vi "SQLHistorylab.vi"() -> ()   [LabVIEW 2013]
uses:
  <vilib>/Platform/TimedLoop/XDataNode/timing_clust.ctl
  <vilib>/Platform/TimedLoop/XDataNode/nitl_modes.ctl
  <vilib>/Platform/TimedLoop/XDataNode/wakeup.ctl
  <vilib>/platform/TimedLoop/XDataNode/XDataNode.xnode
  <vilib>/Platform/TimedLoop/XDataNode/XDNodeRunTimeDep.lvlib
panel:
  out "SSE PV":string
  out "BL13-2SPECPV":string
  out "HIROHITO1PC":T1(plugin-control)
  out "BL13-2DVMPV":string
  out "decimal integer string":string
  out "time string":string
  out "date string":string
  out "CAM2":T1(plugin-control)
  out "CAM1":T1(plugin-control)
  out "CAM3":T1(plugin-control)
  in  "13-2SPEC PV":bool
  out "PV2ELOG":string
  in  "Author":string
  in  "Subject":string
  out "concatenated string":string
  out "standard error":string
  out "standard output":string
  in  "Path":path
  in  "Logbook":u16(ring) items=["BL13-2", "BL13-2 APPES", "BL13-2 SSE"]
  in  "Attachment":bool
  in  "Cam5":bool
  in  "Cam4":bool
  in  "Cam3":bool
  in  "Cam2":bool
  in  "Cam1":bool
  in  "R3000/XES PV":bool
  in  "SES-100PV":bool
  in  "SSE PV":bool
  in  "APPES  PV":bool
  in  "13-2DVM PV":bool
  in  "Submit":bool
  in  "stop":bool
  in  "ELOG":string
  # "BL13-2 ELOG"
  # "[PV name] [PV value] [Time]"
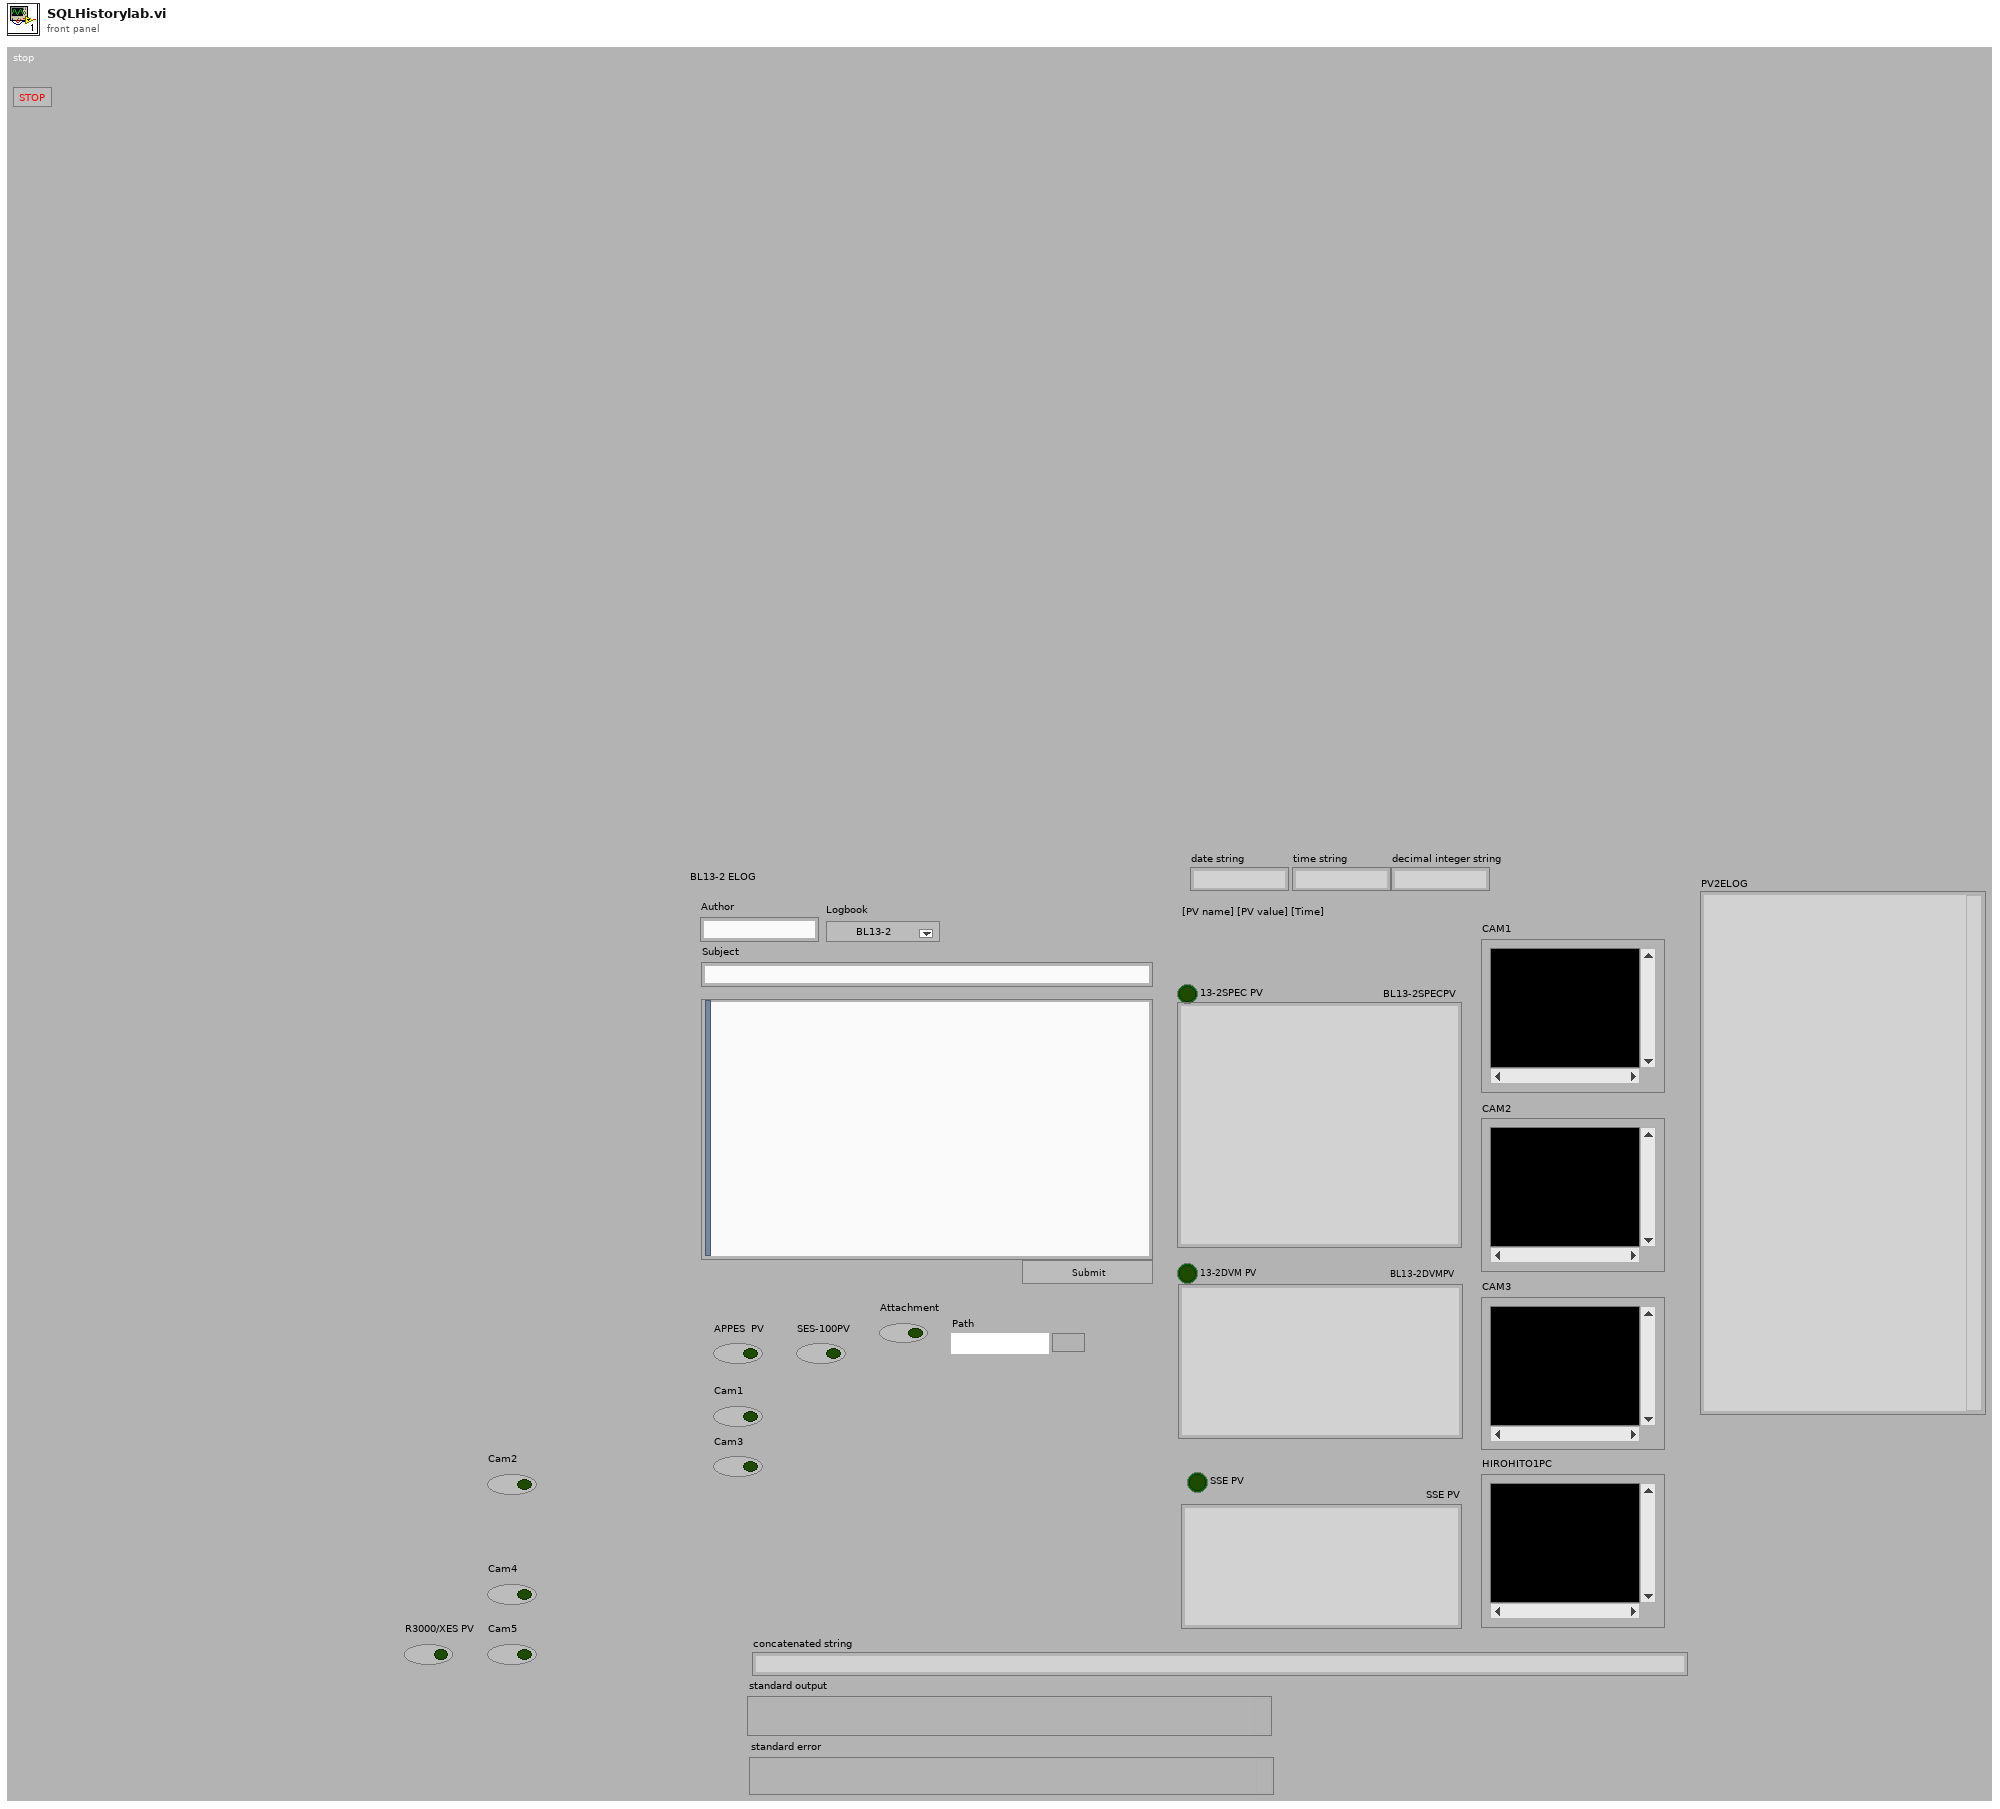
[diagram p1: front panel]
types:
  T1 = typedef "IMAQ Image.ctl" = refnum<image>
  T2 = typedef "XDNodeRunTimeDep.lvlib/timing_clust.ctl" = cluster{"Expected End [f-1]":u64, "Actual End [f-1]":u64, "Finished Late? [f-1]":bool, "Expected End [i-1]":u64, "Actual End [i-1]":u64, "Finished Late? [i-1]":bool, "Expected Start [i]":u64, "Actual Start [i]":u64, "Expected Start [f]":u64, "Actual Start [f]":u64, "Source Name":string, "Structure Name":string, "Period":i64, "Deadline":i64, "Offset":i64, "Start":i64, "Priority":i32, "Timeout":i32, "Mode":T3, "Wakeup Reason":T4, "Error":errorcluster, "Source Type":string, "Secondary Source Type":string, "Global End Time":u64, "Global Start Time":u64, "Frame Duration":u64, "Iteration Duration":u64, "Assigned CPU":i32, "I/O Scan Engine Mode":u32}
  T3 = typedef "XDNodeRunTimeDep.lvlib/nitl_modes.ctl" = enum32{"No Change", "Process missed periods, maintain original phase", "Discard missed periods, maintain original phase", "Process missed periods, ignore original phase", "Discard missed periods, ignore original phase"}
  T4 = typedef "XDNodeRunTimeDep.lvlib/wakeup.ctl" = enum32{"Normal", "Aborted", "Asynchronous wakeup", "Timing source error", "Timed loop error", "Timeout"}
  T5 = enum16{"open", "replace", "create", "open or create", "replace or create", "replace or create with confirmation"}
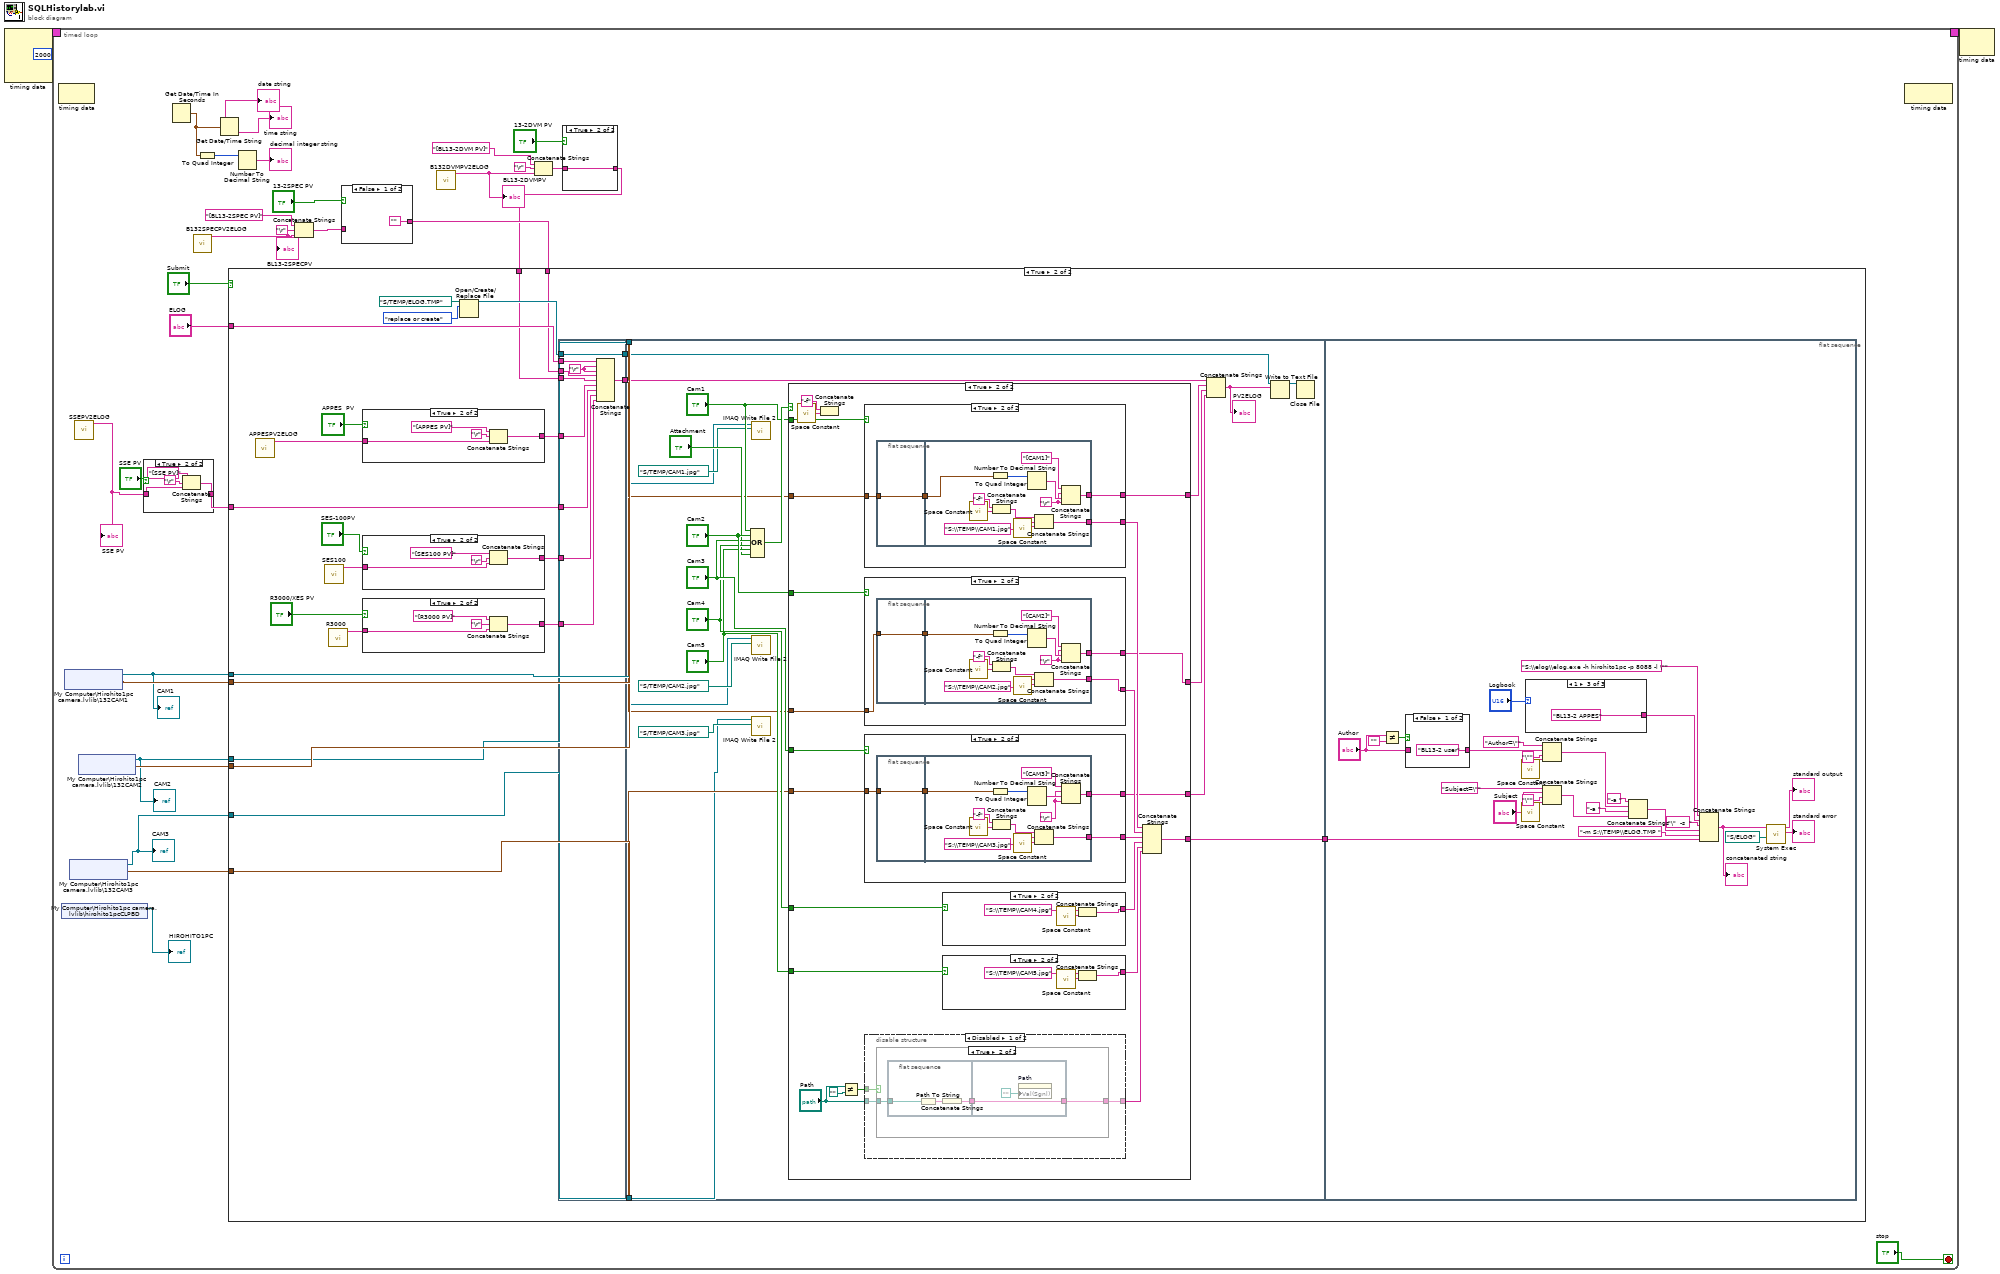
[diagram p0: block diagram]
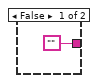
[diagram p2: hidden frame]
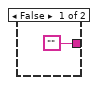
[diagram p3: hidden frame]
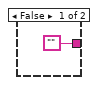
[diagram p6: hidden frame]
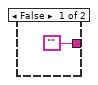
[diagram p7: hidden frame]
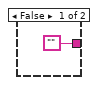
[diagram p8: hidden frame]
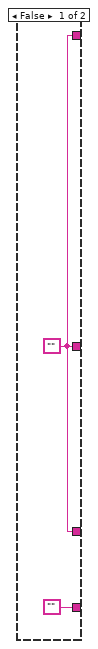
[diagram p9: hidden frame]
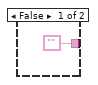
[diagram p10: hidden frame]
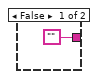
[diagram p12: hidden frame]
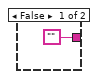
[diagram p13: hidden frame]
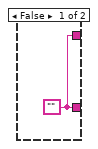
[diagram p14: hidden frame]
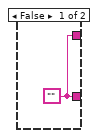
[diagram p15: hidden frame]
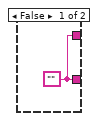
[diagram p16: hidden frame]
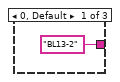
[diagram p18: hidden frame]
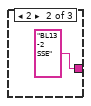
[diagram p19: hidden frame]
diagram:
  n1 = node-c288(i64 2000 ("Period")) -> (w3:T2)  [unwired: 3 in]
  n2 = timed-loop {
    timing: w3 -> [_]
    timing-out: [_] -> w2
    stop <- "stop" stop-if-true
    n3 = node-c288() -> ()  [unwired: 1 in, 1 out]
    n4 = shared-variable "My Computer\\Hirohito1pc camera.lvlib\\hirohito1pcCLPBD"() -> (→"HIROHITO1PC":refnum<image>)  [unwired: 1 in, 1 out]
    n5 = shared-variable "My Computer\\Hirohito1pc camera.lvlib\\132CAM1"() -> (w13:refnum<image>, w14:timestamp)  [unwired: 1 in, 1 out]
    "CAM1" <- w13
    n6 = shared-variable "My Computer\\Hirohito1pc camera.lvlib\\132CAM3"() -> (w9:refnum<image>, w10:timestamp)  [unwired: 1 in, 1 out]
    "CAM3" <- w9
    n7 = call "SSEPV2ELOG.vi"() -> ("concatenated string"=w4:string)  [unwired: 11 in]
    "SSE PV" <- w4
    n8 = shared-variable "My Computer\\Hirohito1pc camera.lvlib\\132CAM2"() -> (w11:refnum<image>, w12:timestamp)  [unwired: 1 in, 1 out]
    "CAM2" <- w11
    n9 = case shown="True" "SSE PV" {
      tunnel: ["" w36] -> w5
      tunnel: w4 -> [_ w37]
      frame False {
      }
      frame True {
        n10 = Concatenate Strings("[SSE PV]" ("string"), "\r", w37) -> (w36:string)
      }
    }
    n11 = Get Date/Time In Seconds() -> (seconds since 1Jan1904=w26:timestamp)
    n12 = call "B132SPECPV2ELOG.vi"() -> ("concatenated string"=w25:string)  [unwired: 11 in]
    "BL13-2SPECPV" <- w25
    n13 = To Quad Integer(1:w26) -> (0:w28:i64)
    n14 = Get Date/Time String(seconds (now)=w26) -> (date string=→"date string":string, time string=→"time string":string)  [unwired: 2 in]
    n15 = Number To Decimal String(number=w28) -> (decimal integer string=→"decimal integer string":string)  [unwired: 1 in]
    n16 = Concatenate Strings("[BL13-2SPEC PV]" ("string"), "\r", w25) -> (w24:string)
    n17 = case shown="False" "13-2SPEC PV" {
      tunnel: ["" w42] -> w20
      tunnel: w24 -> [_ w42]
      frame False {
      }
      frame True {
      }
    }
    n18 = call "B132DVMPV2ELOG.vi"() -> ("concatenated string 2"=w7:string)  [unwired: 11 in]
    "BL13-2DVMPV" <- w7
    n19 = Concatenate Strings("[BL13-2DVM PV]" ("string"), "\r", w7) -> (w19:string)
    n20 = case shown="True" "13-2DVM PV" {
      tunnel: ["" w40] -> w15
      tunnel: w19 -> [_ w40]
      frame False {
      }
      frame True {
      }
    }
    n21 = case shown="True" "Submit" {
      tunnel: "ELOG" -> [_ w69]
      tunnel: w20 -> [_ w53]
      tunnel: w15 -> [_ w52]
      tunnel: w14 -> [_ w51]
      tunnel: w13 -> [_ w50]
      tunnel: w12 -> [_ w49]
      tunnel: w11 -> [_ w48]
      tunnel: w10 -> [_ w47]
      tunnel: w9 -> [_ w46]
      tunnel: w5 -> [_ w45]
      frame False {
      }
      frame True {
        n22 = call "APPESPV2ELOG.vi"() -> ("concatenated string"=w56:string)  [unwired: 11 in]
        n23 = call "SES100.vi"() -> ("text"=w55:string)  [unwired: 11 in]
        n24 = call "R3000.vi"() -> ("text"=w54:string)  [unwired: 11 in]
        n25 = case shown="True" "APPES  PV" {
          tunnel: ["" w82] -> w65
          tunnel: w56 -> [_ w81]
          frame False {
          }
          frame True {
            n26 = Concatenate Strings("[APPES PV]" ("string"), "\r", w81) -> (w82:string)
          }
        }
        n27 = case shown="True" "SES-100PV" {
          tunnel: ["" w79] -> w61
          tunnel: w55 -> [_ w76]
          frame False {
          }
          frame True {
            n28 = Concatenate Strings("[SES100 PV]" ("string"), "\r", w76) -> (w79:string)
          }
        }
        n29 = case shown="True" "R3000/XES PV" {
          tunnel: ["" w74] -> w60
          tunnel: w54 -> [_ w71]
          frame False {
          }
          frame True {
            n30 = Concatenate Strings("[R3000 PV]" ("string"), "\r", w71) -> (w74:string)
          }
        }
        n31 = Open/Create/Replace File(file path (use dialog)=path "S:/TEMP/ELOG.TMP", operation (0:open)=T5."replace or create") -> (refnum out=w66:refnum<file>)  [unwired: 4 in, 2 out]
        n32 = flat-sequence {
          tunnel: w66 -> [w92]
          tunnel: w69 -> [w94]
          tunnel: w52 -> [w89]
          tunnel: w65 -> [w85]
          tunnel: w45 -> [w88]
          tunnel: w61 -> [w87]
          tunnel: w60 -> [w86]
          tunnel: w53 -> [w90]
          tunnel: [w92] -> w59
          tunnel: [w91] -> w58
          tunnel: w59 -> [w95]
          tunnel: w58 -> [w108]
          tunnel: [w105] -> w57
          tunnel: w51 -> [w101]
          tunnel: w50 -> [w100]
          tunnel: w49 -> [w99]
          tunnel: w48 -> [w98]
          tunnel: w47 -> [w97]
          tunnel: w46 -> [w96]
          tunnel: w57 -> [w220]
          frame #0 {
            w93 = "\r"
            n33 = Concatenate Strings(w94, w93, w93, w90, w89, w85, w88, w87, w86) -> (w91:string)
          }
          frame #1 {
            n34 = Compound Arithmetic op=OR("Cam1", "Cam2", "Cam3", "Cam4", "Cam5", "Attachment") -> (w118:bool)
            n35 = call-poly "IMAQ Write File 2"("File Path"=path "S:/TEMP/CAM1.jpg", "Image"=w100) -> ()  [unwired: 8 in, 2 out]
            n36 = call-poly "IMAQ Write File 2"("File Path"=path "S:/TEMP/CAM2.jpg", "Image"=w98) -> ()  [unwired: 8 in, 2 out]
            n37 = call-poly "IMAQ Write File 2"("File Path"=path "S:/TEMP/CAM3.jpg", "Image"=w96) -> ()  [unwired: 8 in, 2 out]
            n38 = case shown="True" w118 {
              tunnel: ["" w131] -> w105
              tunnel: "Cam1" -> [_ w136]
              tunnel: "Cam2" -> [_ w135]
              tunnel: "Cam3" -> [_ w134]
              tunnel: "Cam4" -> [_ w133]
              tunnel: "Cam5" -> [_ w132]
              tunnel: [w119 w129] -> w109
              tunnel: [w119 w128] -> w107
              tunnel: [w119 w127] -> w106
              tunnel: w101 -> [_ w123]
              tunnel: w99 -> [_ w122]
              tunnel: w97 -> [_ w121]
              frame False {
                w119 = ""
              }
              frame True {
                n39 = call <vilib>:"Space Constant.vi"() -> ("String"=w142:string)
                n40 = Concatenate Strings("-f", w142) -> ()  [unwired: 1 out]
                n41 = Not Equal?(x="Path", y=path "") -> (x != y?=w125:bool)
                n42 = case shown="True" w136 {
                  tunnel: [w200 w204] -> w141
                  tunnel: [w200 w203] -> w128
                  tunnel: w123 -> [_ w202]
                  frame False {
                    w200 = ""
                  }
                  frame True {
                    n43 = flat-sequence {
                      tunnel: w202 -> [w205]
                      tunnel: [w205] -> w201
                      tunnel: [w215] -> w204
                      tunnel: [w209] -> w203
                      tunnel: w201 -> [w210]
                      frame #0 {
                      }
                      frame #1 {
                        w211 = "\r"
                        n44 = call <vilib>:"Space Constant.vi"() -> ("String"=w207:string)
                        n45 = To Quad Integer(1:w210) -> (0:w214:i64)
                        n46 = Concatenate Strings("-f", w207) -> (w206:string)
                        n47 = call <vilib>:"Space Constant.vi"() -> ("String"=w216:string)
                        n48 = Number To Decimal String(number=w214) -> (decimal integer string=w212:string)  [unwired: 1 in]
                        n49 = Concatenate Strings(w206, "S:\\TEMP\\CAM1.jpg", w216) -> (w215:string)
                        n50 = Concatenate Strings("[CAM1]" ("string"), w211, w212, w211) -> (w209:string)
                      }
                    }
                  }
                }
                n51 = case shown="True" w135 {
                  tunnel: [w182 w186] -> w140
                  tunnel: [w182 w185] -> w127
                  tunnel: w122 -> [_ w184]
                  frame False {
                    w182 = ""
                  }
                  frame True {
                    n52 = flat-sequence {
                      tunnel: w184 -> [w187]
                      tunnel: [w187] -> w183
                      tunnel: [w197] -> w186
                      tunnel: [w191] -> w185
                      tunnel: w183 -> [w194]
                      frame #0 {
                      }
                      frame #1 {
                        w192 = "\r"
                        n53 = call <vilib>:"Space Constant.vi"() -> ("String"=w189:string)
                        n54 = To Quad Integer(1:w194) -> (0:w195:i64)
                        n55 = Concatenate Strings("-f", w189) -> (w188:string)
                        n56 = call <vilib>:"Space Constant.vi"() -> ("String"=w198:string)
                        n57 = Number To Decimal String(number=w195) -> (decimal integer string=w193:string)  [unwired: 1 in]
                        n58 = Concatenate Strings(w188, "S:\\TEMP\\CAM2.jpg", w198) -> (w197:string)
                        n59 = Concatenate Strings("[CAM2]" ("string"), w192, w193, w192) -> (w191:string)
                      }
                    }
                  }
                }
                n60 = case shown="True" w134 {
                  tunnel: [w164 w168] -> w139
                  tunnel: [w164 w167] -> w129
                  tunnel: w121 -> [_ w166]
                  frame False {
                    w164 = ""
                  }
                  frame True {
                    n61 = flat-sequence {
                      tunnel: w166 -> [w169]
                      tunnel: [w169] -> w165
                      tunnel: [w180] -> w168
                      tunnel: [w173] -> w167
                      tunnel: w165 -> [w177]
                      frame #0 {
                      }
                      frame #1 {
                        w174 = "\r"
                        n62 = call <vilib>:"Space Constant.vi"() -> ("String"=w171:string)
                        n63 = To Quad Integer(1:w177) -> (0:w178:i64)
                        n64 = Concatenate Strings("-f", w171) -> (w170:string)
                        n65 = call <vilib>:"Space Constant.vi"() -> ("String"=w181:string)
                        n66 = Number To Decimal String(number=w178) -> (decimal integer string=w175:string)  [unwired: 1 in]
                        n67 = Concatenate Strings(w170, "S:\\TEMP\\CAM3.jpg", w181) -> (w180:string)
                        n68 = Concatenate Strings("[CAM3]" ("string"), w174, w175, w174) -> (w173:string)
                      }
                    }
                  }
                }
                n69 = disable-structure shown="Disabled" {
                  disable-tunnel: [w146 _] -> w130
                  disable-tunnel: w125 -> [w145 _]
                  disable-tunnel: "Path" -> [w144 _]
                  frame Disabled {
                    n70 = case shown="True" w145 {
                      tunnel: w144 -> [_ w150]
                      tunnel: ["" w149] -> w146
                      frame False {
                      }
                      frame True {
                        n71 = flat-sequence {
                          tunnel: w150 -> [w153]
                          tunnel: [w151] -> w148
                          tunnel: [w155] -> w149
                          tunnel: w148 -> [w155]
                          frame #0 {
                            n72 = Path To String(path=w153) -> (string=w152:string)
                            n73 = Concatenate Strings(w152) -> (w151:string)
                          }
                          frame #1 {
                            n74 = property on="Path" class="Path"("Val(Sgnl)"=path "") -> ()  [unwired: 2 in, 2 out]
                          }
                        }
                      }
                    }
                  }
                  frame Enabled {
                  }
                }
                n75 = case shown="True" w133 {
                  tunnel: ["" w161] -> w138
                  frame False {
                  }
                  frame True {
                    n76 = call <vilib>:"Space Constant.vi"() -> ("String"=w162:string)
                    n77 = Concatenate Strings("S:\\TEMP\\CAM4.jpg", w162) -> (w161:string)
                  }
                }
                n78 = case shown="True" w132 {
                  tunnel: ["" w157] -> w137
                  frame False {
                  }
                  frame True {
                    n79 = call <vilib>:"Space Constant.vi"() -> ("String"=w158:string)
                    n80 = Concatenate Strings("S:\\TEMP\\CAM5.jpg", w158) -> (w157:string)
                  }
                }
                n81 = Concatenate Strings(w141, w140, w139, w138, w137, w130) -> (w131:string)
              }
            }
            n82 = Concatenate Strings(w108, w107, w106, w109) -> (w110:string)
            "PV2ELOG" <- w110
            n83 = Write to Text File(file (use dialog)=w95, text=w110) -> (refnum out=w111:refnum<file>)  [unwired: 2 in, 2 out]
            n84 = Close File(refnum=w111) -> ()  [unwired: 1 in, 2 out]
          }
          frame #2 {
            n85 = Not Equal?(x="Author", y="") -> (x != y?=w229:bool)
            n86 = case shown="False" w229 {
              tunnel: "Author" -> [_ w245]
              tunnel: ["BL13-2 user" w245] -> w235
              frame False {
              }
              frame True {
              }
            }
            n87 = call <vilib>:"Space Constant.vi"() -> ("String"=w238:string)
            n88 = call <vilib>:"Space Constant.vi"() -> ("String"=w237:string)
            n89 = case shown="1" "Logbook" {
              tunnel: ["BL13-2" "BL13-2 SSE" "BL13-2 APPES"] -> w218
              frame 0, Default {
              }
              frame 2 {
              }
              frame 1 {
              }
            }
            n90 = Concatenate Strings("Author=\"" ("string"), w235, "\"" ("string"), w238) -> (w240:string)
            n91 = Concatenate Strings("Subject=\"" ("string"), "Subject", "\"" ("string"), w237) -> (w242:string)
            n92 = Concatenate Strings("-a ", w240, "-a " ("string"), w242) -> (w241:string)
            n93 = Concatenate Strings("S:\\elog\\elog.exe -h hirohito1pc -p 8088 -l \"" ("command line"), w218, "\"  -s  " ("command line"), w241, "-m S:\\TEMP\\ELOG.TMP " ("string"), w220) -> (w224:string)
            "concatenated string" <- w224
            n94 = call <vilib>:"System Exec.vi"("working directory"=path "S:/ELOG", "command line"=w224) -> ("standard error"=→"standard error":string, "standard output"=→"standard output":string)  [unwired: 6 in, 2 out]
          }
        }
      }
    }
    n95 = node-c288() -> ()  [unwired: 1 in, 1 out]
  }
  n96 = node-c288(w2) -> ()  [unwired: 1 out]
